vi "file2FIR.vi"(6 "Reset":bool, 9 "file path (use dialog)":path=path "c:/bob.dat", 11 "signal in":dbl) -> (3 "signal out":dbl)   [LabVIEW 2010, in "kevLib2011.lvlib"]
uses:
  kevLib2011.lvlib
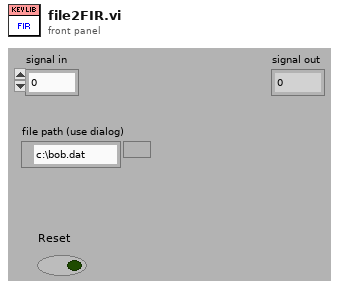
[diagram p1: front panel]
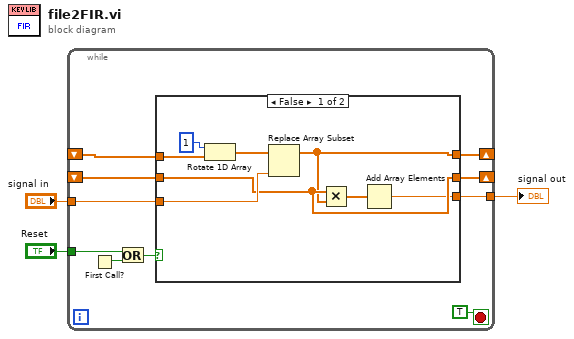
[diagram p0: block diagram]
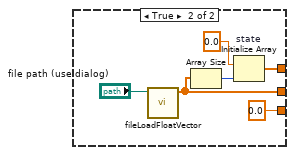
[diagram p2: hidden frame]
diagram:
  n1 = while {
    tunnel: "signal in" -> [w7]
    tunnel: "Reset" -> [w10]
    shift-right: [w5] -> _
    shift-left: _ -> [w8]
    shift-right: [w9] -> _
    shift-left: _ -> [w6]
    tunnel: [w4] -> w1
    stop <- TRUE stop-if-true
    n2 = First Call?() -> (First Call?: T/F=w12:bool)
    n3 = Or(x=w10, y=w12) -> (x .or. y?=w11:bool)
    n4 = case shown="False" w11 {
      tunnel: [w16 w24] -> w5
      tunnel: [w17 w23] -> w9
      tunnel: w8 -> [w20 _]
      tunnel: w7 -> [w19 _]
      tunnel: w6 -> [w17 _]
      tunnel: [w14 0.0] -> w4
      frame False {
        n5 = Rotate 1D Array(1:w20, 2:1 ("n")) -> (0:w18:dbl[])
        n6 = Replace Array Subset(array=w18, new element=w19) -> (w16:dbl[])  [unwired: 1 in]
        n7 = Multiply(x=w17, y=w16) -> (x*y=w15:dbl[])
        n8 = Add Array Elements(numeric array=w15) -> (sum=w14:dbl)
      }
      frame True {
        n9 = call "fileLoadFloatVector.vi"("File Path"="file path (use dialog)") -> ("Float Vector"=w23:dbl[])  [unwired: 9 in, 1 out]
        n10 = Array Size(array=w23) -> (size(s)=w26:i32)
        n11 = Initialize Array "state"(0.0 ("element"), w26) -> (w24:dbl[])
      }
    }
  }
  "signal out" <- w1
